vi "CANOpen_SDO Write RW.vi"(8 "error in":errorcluster, 11 "SDO Asynch in":T1 {"HW Dyn Read"."Resp Chan."."Chan Refs" format="%.0x"; "HW Dyn Read"."Req Chan."."Chan Refs" format="%.0x"; "HW Dyn Write"."Resp Chan."."Chan Refs" format="%.0x"; "HW Dyn Write"."Req Chan."."Chan Refs" format="%.0x"; "List SDO"."Resp Chan."."Chan Refs" format="%.0x"; "List SDO"."Req Chan."."Chan Refs" format="%.0x"}) -> (0 "error out":errorcluster, 3 "SDO Asynch out":T1 {"HW Dyn Read"."Resp Chan."."Chan Refs" format="%.0x"; "HW Dyn Read"."Req Chan."."Chan Refs" format="%.0x"; "HW Dyn Write"."Resp Chan."."Chan Refs" format="%.0x"; "HW Dyn Write"."Req Chan."."Chan Refs" format="%.0x"; "List SDO"."Resp Chan."."Chan Refs" format="%.0x"; "List SDO"."Req Chan."."Chan Refs" format="%.0x"})   [LabVIEW 2013, in "CANOpen Addon Custom Device.lvlib"]
uses:
  CANOpen Addon Custom Device.lvlib
  CANOpen_VS SDOs Data Refs.ctl
  <vilib>/NI Veristand/Custom Device API/Data Reference.ctl
  Async VIs/CANOpen_Main/SubVIs/CanOpen_SDO Dynamic queue.ctl
  Shared Code/CANOpen_SDO queue W data.ctl
  Shared Code/CANOpen_SDO queue mode.ctl
  Shared Code/CANOpen_PDO Data Type in queue.ctl
  <vilib>/NI Veristand/Custom Device API/Global Data Refs.vi
  <vilib>/NI Veristand/Custom Device API/Custom Device API.lvlib
  Debug/SubVIs/Global debug.vi
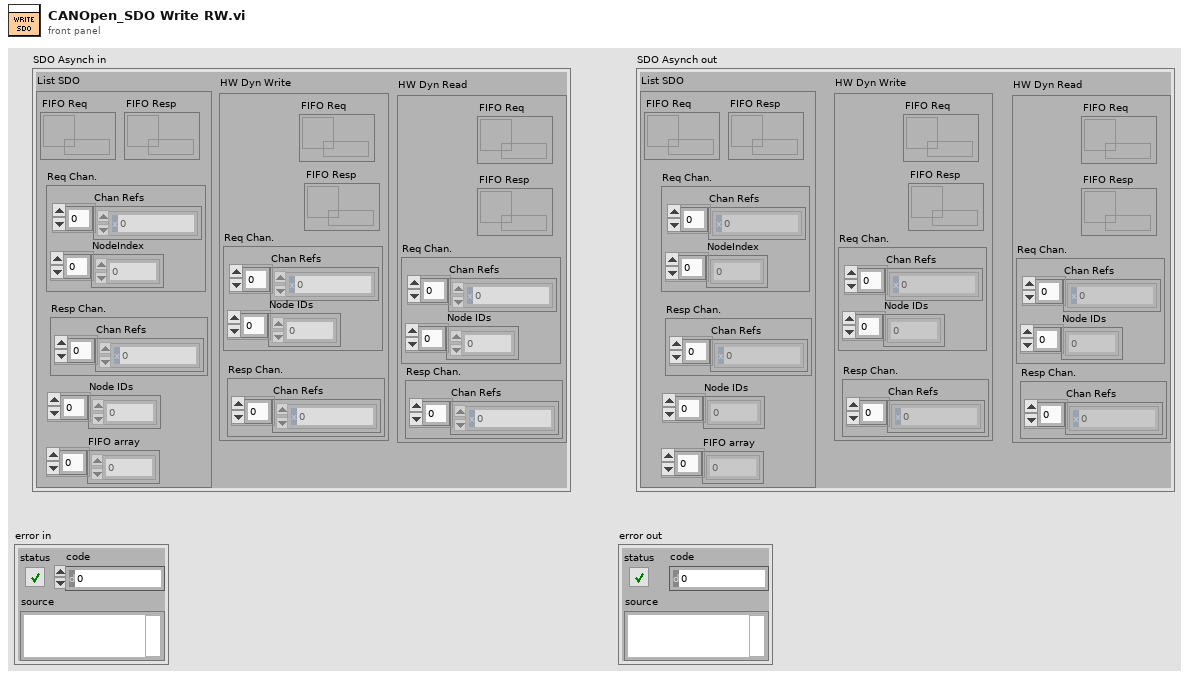
[diagram p1: front panel]
types:
  T1 = typedef "CANOpen Addon Custom Device.lvlib/CANOpen_VS SDOs Data Refs.ctl" = cluster{"List SDO":cluster{"FIFO Req":refnum<k33>, "Req Chan.":cluster{"Chan Refs":T2[], "NodeIndex":dbl[]}, "FIFO Resp":refnum<k33>, "Resp Chan.":cluster{"Chan Refs":T2[]}, "Node IDs":u8[], "FIFO array":dbl[]}, "HW Dyn Write":cluster{"FIFO Req":refnum<k33>, "FIFO Resp":refnum<k33>, "Req Chan.":cluster{"Chan Refs":T2[], "Node IDs":u8[]}, "Resp Chan.":cluster{"Chan Refs":T2[]}}, "HW Dyn Read":cluster{"FIFO Req":refnum<k33>, "FIFO Resp":refnum<k33>, "Req Chan.":cluster{"Chan Refs":T2[], "Node IDs":u8[]}, "Resp Chan.":cluster{"Chan Refs":T2[]}}}
  T2 = typedef "Custom Device API.lvlib/Data Reference.ctl" = i32
  T3 = typedef "CANOpen Addon Custom Device.lvlib/CANOpen_SDO queue mode.ctl" = enum16{"WRITE write", "WRITE response", "READ write", "READ response"}
  T4 = typedef "CANOpen Addon Custom Device.lvlib/CanOpen_SDO Dynamic queue.ctl" = cluster{"Node ID":u8, "Data":T5}
  T5 = typedef "CANOpen Addon Custom Device.lvlib/CANOpen_SDO queue W data.ctl" = cluster{"Object Index":u16, "Object Sub-Index (0)":u8, "Mode":T3, "Data Type":T6, "Value":dbl, "Status code":dbl, "Byte Order":enum16{"big-endian, network order", "little-endian"}}
  T6 = typedef "CANOpen Addon Custom Device.lvlib/CANOpen_PDO Data Type in queue.ctl" = enum16{"U8", "U16", "U32", "I8", "I16", "I32", "Single", "Double"}
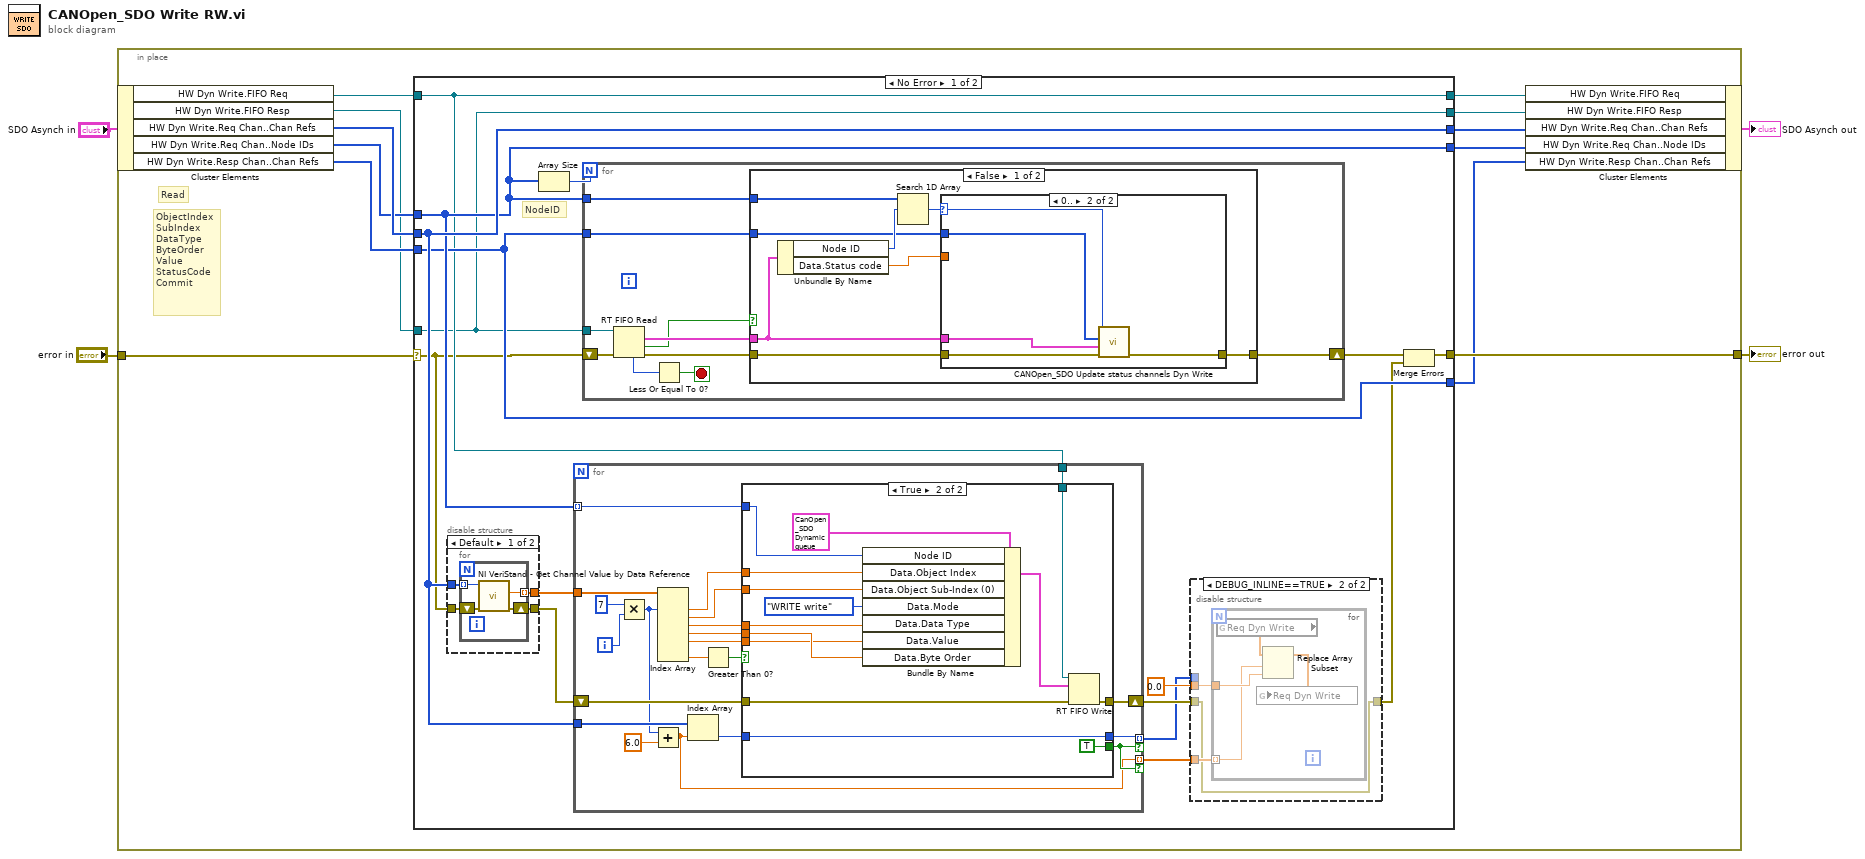
[diagram p0: block diagram]
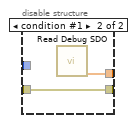
[diagram p4: hidden frame]
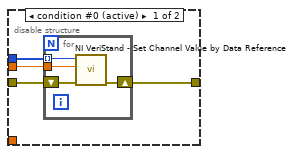
[diagram p5: hidden frame]
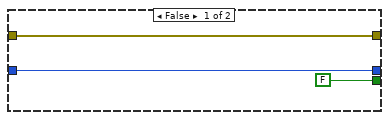
[diagram p6: hidden frame]
diagram:
  n1 = in-place {
    in-place-border: "error in" -> [w13]
    in-place-border: [w12] -> w1
    # "Read"
    # "ObjectIndex\nSubIndex\nDataType\nByteOrder\nValue\nStatusCode\nCommit"
    n2 = in-place-cluster #1("SDO Asynch in") -> ("HW Dyn Write.FIFO Req"=w6:refnum<k33>, "HW Dyn Write.FIFO Resp"=w5:refnum<k33>, "HW Dyn Write.Req Chan..Chan Refs"=w15:T2[], "HW Dyn Write.Req Chan..Node IDs"=w7:u8[], "HW Dyn Write.Resp Chan..Chan Refs"=w11:T2[])
    n3 = case shown="No Error" w13 {
      selector: w13 -> [w17 w122]
      tunnel: [w28 w122] -> w12
      tunnel: w5 -> [w18 w126]
      tunnel: [w18 w126] -> w16
      tunnel: w15 -> [w31 w125]
      tunnel: w7 -> [w30 w124]
      tunnel: [w31 w125] -> w14
      tunnel: [w30 w124] -> w8
      tunnel: w6 -> [w21 w123]
      tunnel: w11 -> [w29 w121]
      tunnel: [w21 w123] -> w10
      tunnel: [w29 w121] -> w9
      frame No Error {
        # "NodeID"
        n4 = disable-structure shown="Default" {
          disable-tunnel: w31 -> [w61 _]
          disable-tunnel: w17 -> [w60 w67]
          disable-tunnel: [w59 w67] -> w25
          disable-tunnel: [w58 w66] -> w26
          frame condition #0 (active) {
            n5 = for {
              tunnel: w61 -> [w65] mode=indexing
              tunnel: [w64] -> w58 mode=indexing
              shift-right: [w62] -> w59
              shift-left: w60 -> [w63]
              n6 = call <vilib>:"NI VeriStand - Get Channel Value by Data Reference.vi"("error in (no error)"=w63, "Data Reference in"=w65) -> ("error out"=w62:errorcluster, "Value"=w64:dbl)  [unwired: 8 in]
            }
          }
          frame condition #1 {
            n7 = call "Read Debug SDO.vi"() -> ("Req Dyn Write"=w66:dbl[])  [unwired: 8 in, 3 out]
          }
        }
        n8 = Array Size(array=w30) -> (size(s)=w19:i32)
        n9 = for {
          tunnel: w30 -> [w84] mode=indexing
          tunnel: w26 -> [w103]
          shift-right: [w93] -> w23
          shift-left: w25 -> [w94]
          tunnel: w31 -> [w92]
          tunnel: [w88] -> w22 mode=indexing if=w85
          tunnel: w21 -> [w87]
          tunnel: [w83] -> w20 mode=indexing if=w85
          i -> [w86]
          n10 = Multiply(x=7, y=w86) -> (x*y=w90:i32)
          n11 = Add(x=w90, y=6.0) -> (x+y=w83:dbl)
          n12 = Index Array(array=w103, index #1=w90) -> (element #1=w99:dbl, element #2=w98:dbl, element #3=w97:dbl, element #4=w96:dbl, element #5=w95:dbl, element #7=w101:dbl)  [unwired: 6 in, 1 out]
          n13 = Index Array(array=w92, index=w83) -> (element=w89:T2)
          n14 = Greater Than 0?(x=w101) -> (x > 0?=w100:bool)
          n15 = case shown="True" w100 {
            tunnel: [w106 w120] -> w93
            tunnel: w84 -> [_ w107]
            tunnel: w99 -> [_ w117]
            tunnel: w98 -> [_ w116]
            tunnel: w97 -> [_ w114]
            tunnel: w96 -> [_ w113]
            tunnel: w95 -> [_ w112]
            tunnel: w94 -> [w106 w111]
            tunnel: w89 -> [w105 w109]
            tunnel: [w105 w109] -> w88
            tunnel: [FALSE TRUE] -> w85
            tunnel: w87 -> [_ w108]
            frame False {
            }
            frame True {
              n16 = Bundle By Name(cluster=T4 {"Node ID"=0, "Data"={"Object Index"=0, "Object Sub-Index (0)"=0, "Mode"=enum."WRITE write", "Data Type"=enum."U8", "Value"=0.0, "Status code"=0.0, "Byte Order"=enum."little-endian"}} ("element"), "Node ID"=w107, "Data.Object Index"=w117, "Data.Object Sub-Index (0)"=w116, "Data.Mode"=CANOpen_SDO_queue_mode."WRITE write", "Data.Data Type"=w114, "Data.Value"=w112, "Data.Byte Order"=w113) -> (w118:T4)
              n17 = RT FIFO Write(0:w108, 1:w118, 3:w111) -> (11:w120:errorcluster)  [unwired: 2 in, 3 out]
            }
          }
        }
        n18 = for {
          N: w19 -> [_]
          tunnel: w30 -> [w38]
          tunnel: w18 -> [w40]
          shift-right: [w35] -> w32
          shift-left: w17 -> [w39]
          tunnel: w29 -> [w37]
          stop <- w41 stop-if-true
          n19 = RT FIFO Read(0:w40, 3:w39) -> (7:w42:u32, 9:w34:T4, 10:w33:bool, 11:w36:errorcluster)  [unwired: 2 in, 1 out]
          n20 = Less Or Equal To 0?(x=w42) -> (x <= 0?=w41:bool)
          n21 = case shown="False" w33 {
            tunnel: w38 -> [w50 _]
            tunnel: w37 -> [w47 _]
            tunnel: w36 -> [w46 w57]
            tunnel: [w45 w57] -> w35
            tunnel: w34 -> [w43 _]
            frame False {
              n22 = Unbundle By Name(w43) -> ("Node ID"=w49:u8, "Data.Status code"=w44:dbl)
              n23 = Search 1D Array(1D array=w50, element=w49) -> (index of element=w48:i32)  [unwired: 1 in]
              n24 = case shown="0.." w48 {
                selector: w48 -> [_ w56]
                tunnel: w47 -> [_ w55]
                tunnel: w46 -> [w51 w54]
                tunnel: [w51 w53] -> w45
                tunnel: w44 -> [_ _]
                tunnel: w43 -> [_ w52]
                frame -1, Default {
                }
                frame 0.. {
                  n25 = call "CANOpen_SDO Update status channels Dyn Write.vi"("error in (no error)"=w54, "Status Data"=w52, "Chan Refs"=w55, "index of element"=w56) -> ("error out"=w53:errorcluster)  [unwired: 7 in]
                }
              }
            }
            frame True {
            }
          }
        }
        n26 = disable-structure shown="DEBUG_INLINE==TRUE" {
          disable-tunnel: [w71 w76] -> w27
          disable-tunnel: w23 -> [w70 w76]
          disable-tunnel: w22 -> [w69 _]
          disable-tunnel: 0.0 ("Value") -> [w68 w78]
          disable-tunnel: w20 -> [_ w77]
          frame condition #0 (active) {
            n27 = for {
              tunnel: w69 -> [w73] mode=indexing
              shift-right: [w74] -> w71
              shift-left: w70 -> [w75]
              tunnel: w68 -> [w72]
              n28 = call <vilib>:"NI VeriStand - Set Channel Value by Data Reference.vi"("error in (no error)"=w75, "Value"=w72, "Data Reference in"=w73) -> ("error out"=w74:errorcluster)  [unwired: 8 in]
            }
          }
          frame condition #1 {
            n29 = for {
              tunnel: w78 -> [w80]
              tunnel: w77 -> [w79] mode=indexing
              n30 = global read "Global debug.vi" "Req Dyn Write"() -> (w81:dbl[])
              n31 = Replace Array Subset(array=w81, new element=w80, index=w79) -> (w82:dbl[])
              n32 = global write "Global debug.vi" "Req Dyn Write"(w82) -> ()
            }
          }
        }
        n33 = Merge Errors(w32, w27) -> (w28:errorcluster)
      }
      frame Error {
      }
    }
    n34 = in-place-cluster #1("HW Dyn Write.FIFO Req"=w10, "HW Dyn Write.FIFO Resp"=w16, "HW Dyn Write.Req Chan..Chan Refs"=w14, "HW Dyn Write.Req Chan..Node IDs"=w8, "HW Dyn Write.Resp Chan..Chan Refs"=w9) -> (→"SDO Asynch out":T1)
  }
  "error out" <- w1
